vi "ImageFacialDetection_Create.vi"(8 "error in (no error)":errorcluster, 9 "Console visibility (hide)":T1=enum."Hide Console", 10 "Path to Python Module (.py File)":path, 11 "reference in":refnum<class "ImageFacialDetection.lvclass">) -> (0 "error out":errorcluster, 3 "reference out":refnum<class "ImageFacialDetection.lvclass">)   [LabVIEW 2017, in "ImageFacialDetection.lvclass"]
uses:
  ImageFacialDetection.lvclass
  <vilib>/Enthought/Python Integration Toolkit/api/Console Visibility.ctl
  <vilib>/Enthought/Python Integration Toolkit/Python Integration Toolkit.lvlib
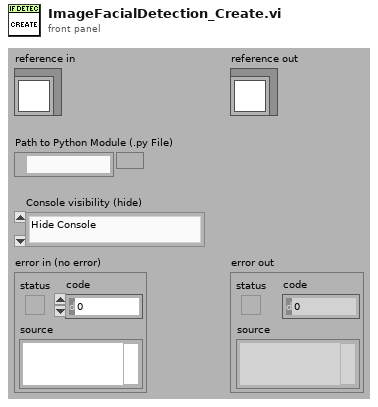
[diagram p1: front panel]
types:
  T1 = typedef "Python Integration Toolkit.lvlib/Console Visibility.ctl" = enum16{"Show Console", "Show Console While Running", "Hide Console"}
  T2 = typedef "Python Integration Toolkit.lvlib/Session ID.ctl" = u64
  T3 = typedef "ImageClassification.lvclass/ObjectAttributes.ctl" = cluster{"Path to Python Module (.py File)":path, "Python Session ID":T2}
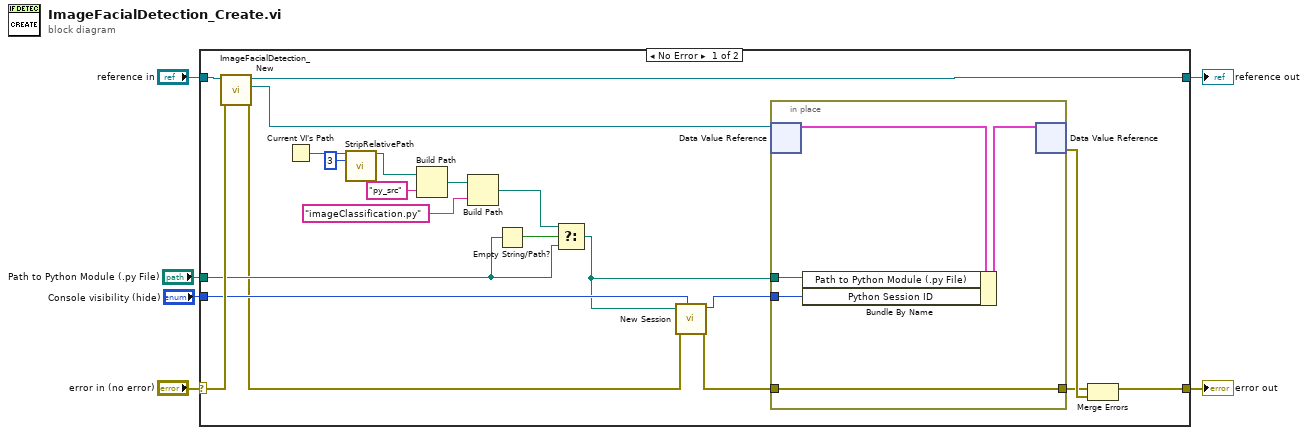
[diagram p0: block diagram]
diagram:
  n1 = case shown="No Error" "error in (no error)" {
    selector: "error in (no error)" -> [w26 w34]
    tunnel: [w23 w34] -> w5
    tunnel: "reference in" -> [w27 w33]
    tunnel: [w25 w33] -> w3
    tunnel: "Path to Python Module (.py File)" -> [w15 _]
    tunnel: "Console visibility (hide)" -> [w11 _]
    frame No Error {
      n2 = call "ImageFacialDetection_New.vi"("error in (no error)"=w26, "reference in"=w27) -> ("error out"=w8:errorcluster, "DVRRefOut"=w22:refnum<data-value>, "reference out"=w25:refnum<class "ImageFacialDetection.lvclass">)  [unwired: 6 in, 1 out]
      n3 = Current VI's Path() -> (path=w14:path)
      n4 = call "StripRelativePath.vi"("URL"=w14, "Levels To Strip"=3) -> ("Stripped URL"=w13:path)  [unwired: 13 in]
      n5 = Build Path(base path=w13, name or relative path="py_src") -> (appended path=w19:path)
      n6 = Build Path(base path=w19, name or relative path="imageClassification.py") -> (appended path=w17:path)
      n7 = Empty String/Path?(string/path=w15) -> (empty?=w16:bool)
      n8 = Select(t=w17, s=w16, f=w15) -> (s? t:f=w9:path)
      n9 = call <vilib>:"New Session.vi"("Console Visibility"=w11, "error in (no error)"=w8, "Path to Python Module (.py File)"=w9) -> ("error out"=w7:errorcluster, "Session ID out"=w10:T2)  [unwired: 7 in]
      n10 = in-place {
        in-place-border: w7 -> [w30]
        in-place-border: [w30] -> w21
        in-place-border: w9 -> [w29]
        in-place-border: w10 -> [w28]
        n11 = in-place-dvr #1(w22) -> (w31:T3)  [unwired: 1 out]
        n12 = Bundle By Name(cluster=w31, "Path to Python Module (.py File)"=w29, "Python Session ID"=w28) -> (w32:T3)
        n13 = in-place-dvr #1(w32) -> (w24:errorcluster)  [unwired: 1 out]
      }
      n14 = Merge Errors(w21, w24) -> (w23:errorcluster)
    }
    frame Error {
      # "VI-TechBaseTemplate_Simple_6x8x6"
    }
  }
  "error out" <- w5
  "reference out" <- w3
